vi "openValveMs.vi"(0 "milliseconds to wait":u32=100, 1 "valve data close":bool[](array[boolean])=[FALSE, TRUE, FALSE, FALSE, FALSE, FALSE, FALSE, FALSE], 2 "valve data open":bool[](array[boolean])=[TRUE, FALSE, FALSE, FALSE, FALSE, FALSE, FALSE, FALSE]) -> ()   [LabVIEW 2011]
uses:
  GlobalDAQ.vi
  <vilib>/ULx/Write.llb/ULx Write (Digital 1D Bool 1Chan 1Samp).vi
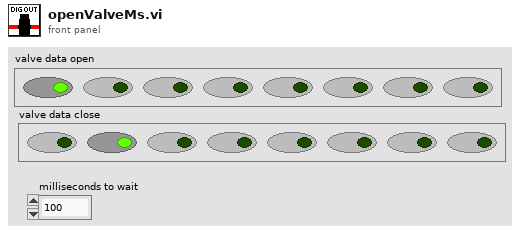
[diagram p1: front panel]
types:
  T1 = typedef "Semaphore RefNum" = refnum<k1>
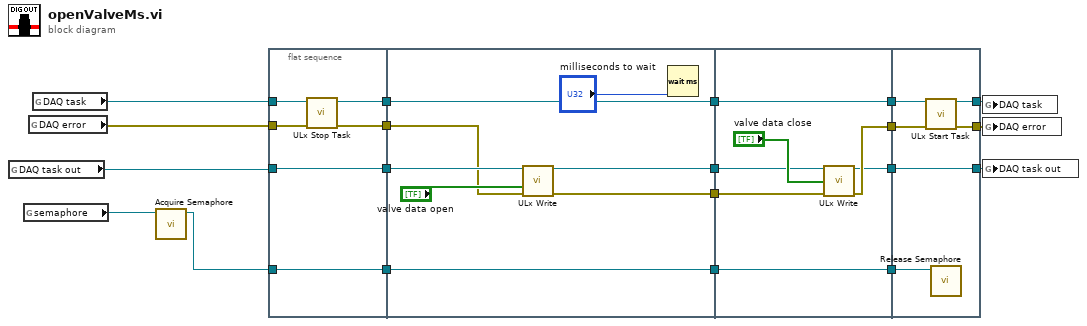
[diagram p0: block diagram]
diagram:
  n1 = global read "GlobalDAQ.vi" "DAQ task out"() -> (w12:refnum<k24>)
  n2 = global read "GlobalDAQ.vi" "semaphore"() -> (w11:T1)
  n3 = global read "GlobalDAQ.vi" "DAQ error"() -> (w17:errorcluster)
  n4 = global read "GlobalDAQ.vi" "DAQ task"() -> (w20:refnum<k24>)
  n5 = call <vilib>:"Acquire Semaphore.vi"("semaphore"=w11) -> ("semaphore out"=w9:T1)  [unwired: 4 in, 2 out]
  n6 = flat-sequence {
    tunnel: w20 -> [w26]
    tunnel: [w25] -> w19
    tunnel: w17 -> [w24]
    tunnel: [w23] -> w16
    tunnel: w12 -> [w23]
    tunnel: [w22] -> w14
    tunnel: [w21] -> w10
    tunnel: w9 -> [w21]
    tunnel: [w34] -> w8
    tunnel: w19 -> [w34]
    tunnel: w16 -> [w33]
    tunnel: [w32] -> w6
    tunnel: w14 -> [w30]
    tunnel: w10 -> [w29]
    tunnel: [w29] -> w4
    tunnel: [w27] -> w2
    tunnel: w8 -> [w41]
    tunnel: [w41] -> w7
    tunnel: w6 -> [w35]
    tunnel: [w37] -> w5
    tunnel: w4 -> [w40]
    tunnel: [w40] -> w3
    tunnel: w2 -> [w38]
    tunnel: [w36] -> w1
    tunnel: w7 -> [w47]
    tunnel: [w46] -> w18
    tunnel: [w42] -> w15
    tunnel: w5 -> [w45]
    tunnel: [w44] -> w13
    tunnel: w3 -> [w43]
    tunnel: w1 -> [w42]
    frame #0 {
      n7 = call <vilib>:"ULx Stop Task.vi"("error in"=w24, "task in"=w26) -> ("error out"=w22:errorcluster, "task out"=w25:refnum<k24>)  [unwired: 8 in]
    }
    frame #1 {
      n8 = call-poly <vilib>:"ULx Write.vi"("task in"=w33, "data"="valve data open", "error in"=w30) -> ("task out"=w32:refnum<k24>, "error out"=w27:errorcluster)  [unwired: 10 in, 1 out]
      n9 = Wait (ms)(milliseconds to wait="milliseconds to wait") -> ()  [unwired: 1 out]
    }
    frame #2 {
      n10 = call-poly <vilib>:"ULx Write.vi"("task in"=w35, "data"="valve data close", "error in"=w38) -> ("task out"=w36:refnum<k24>, "error out"=w37:errorcluster)  [unwired: 10 in, 1 out]
    }
    frame #3 {
      n11 = call <vilib>:"ULx Start Task.vi"("task in"=w47, "error in"=w45) -> ("task out"=w46:refnum<k24>, "error out"=w44:errorcluster)  [unwired: 12 in]
      n12 = call <vilib>:"Release Semaphore.vi"("semaphore"=w43) -> ()  [unwired: 5 in, 2 out]
    }
  }
  n13 = global write "GlobalDAQ.vi" "DAQ task"(w18) -> ()
  n14 = global write "GlobalDAQ.vi" "DAQ error"(w13) -> ()
  n15 = global write "GlobalDAQ.vi" "DAQ task out"(w15) -> ()
